vi "Interpolate_dBm.vi"() -> ()   [LabVIEW 2018]
panel:
  out "dBm":dbl
  in  "PeakAmplitude":dbl
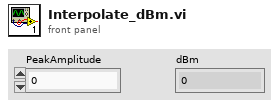
[diagram p1: front panel]
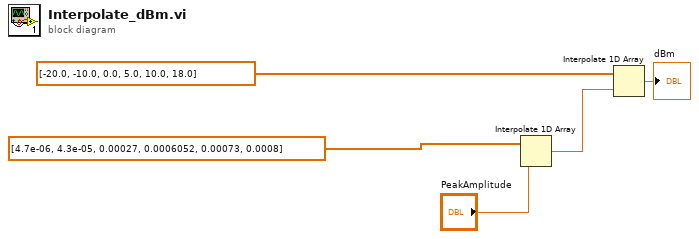
[diagram p0: block diagram]
diagram:
  n1 = Interpolate 1D Array(1:"PeakAmplitude", 2:dbl[] [4.7e-06, 4.3e-05, 0.00027, 0.0006052, 0.00073, 0.0008] ("array of numbers or points")) -> (0:w2:dbl)
  n2 = Interpolate 1D Array(1:w2, 2:dbl[] [-20.0, -10.0, 0.0, 5.0, 10.0, 18.0] ("array of numbers or points")) -> (0:→"dBm":dbl)
